vi "Read MotionCorrectionData.vi"(8 "error in (no error)":errorcluster, 10 "ReadSize":u32, 11 "AODAcq in":refnum<class "AODAcq.lvclass">) -> (0 "error out":errorcluster, 2 "MotionCorrectionData":waveform(i32)[](array[waveform]), 3 "AODAcq out":refnum<class "AODAcq.lvclass">)   [LabVIEW 2014, in "AODAcq.lvclass"]
uses:
  AODAcq.lvclass
  AODAcq.lvclass/AODAcq.ctl
  <vilib>/Utility/error.llb/Error Cluster From Error Code.vi
  <vilib>/rvi/errors/niLvFpgaAdjustHostInterfaceError.vi
  HDF5Tools/LabView/Append To Dataset 2D Double.vi
  <vilib>/rvi/interface/nirviMethod/nirviMethod.xnode
  FPGA_Control/AODRef.ctl
  FPGA Bitfiles/AodScanner_FPGATarget_AODControl(FPGA)_TyJc9yYmyGA.lvbitx
  <vilib>/FPGAPlugInAG/PXIe-7965R/niLvFpga_ReadFifo_PXIe-7965R.vi
  <vilib>/rvi/errors/niLvFpgaMergeErrorWithErrorCode.vi
  HDF5Tools/LabView/HDF5Tools.lvlib
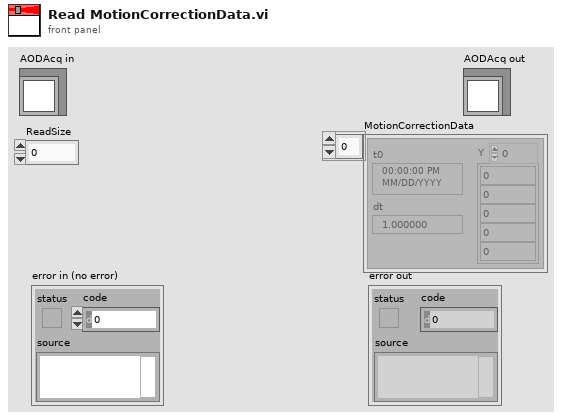
[diagram p1: front panel]
types:
  T1 = typedef "AODRef.ctl" = refnum<k20>
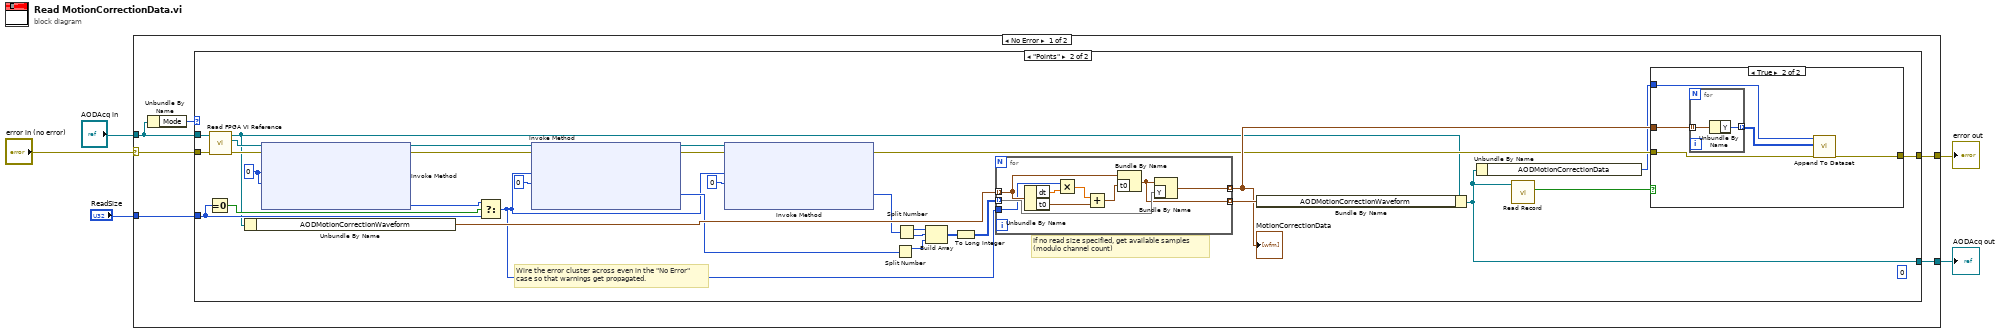
[diagram p0: block diagram]
diagram:
  n1 = case shown="No Error" "error in (no error)" {
    selector: "error in (no error)" -> [w11 w63]
    tunnel: [w8 w63] -> w4
    tunnel: [w9 w62] -> w2
    tunnel: "AODAcq in" -> [w7 w62]
    tunnel: "ReadSize" -> [w10 _]
    frame No Error {
      n2 = Unbundle By Name(w7) -> ("Mode"=w6:enum16{"Idle", "Points", "Volume"})
      n3 = case shown="\"Points\"" w6 {
        tunnel: w7 -> [w13 w44]
        tunnel: w11 -> [w12 w40]
        tunnel: w10 -> [_ w37]
        tunnel: [w13 w32] -> w9
        tunnel: [w12 w31] -> w8
        frame "Idle", Default {
        }
        frame "Points" {
          (unwired) u32 0 ("y")
          w43 = u32 0 ("Number of Elements")
          # "If no read size specified, get available samples \n(modulo channel count)"
          # "Wire the error cluster across even in the \"No Error\"\ncase so that warnings get propagated."
          n4 = Equal To 0?(x=w37) -> (x = 0?=w42:bool)
          n5 = call-dynamic "Read FPGA VI Reference.vi"("error in (no error)"=w40, "AODAcq in"=w44) -> ("error out"=w34:errorcluster, "FPGA VI Reference"=w35:T1, "AODAcq out"=w15:refnum<class "AODAcq.lvclass">)  [unwired: 7 in]
          n6 = Unbundle By Name(w15) -> ("AODMotionCorrectionWaveform"=w39:waveform(i32)[])
          n7 = xnode "Invoke Method"("FPGA VI Reference In"=w35, "error in"=w34, "Number of Elements"=w43, "Timeout (ms)"=w43) -> ("FPGA VI Reference Out"=w27:T1, "error out"=w26:errorcluster, "Elements Remaining"=w36:u32)  [unwired: 1 out]
          n8 = Select(t=w36, s=w42, f=w37) -> (s? t:f=w28:u32)
          n9 = xnode "Invoke Method"("FPGA VI Reference In"=w27, "error in"=w26, "Number of Elements"=w28, "Timeout (ms)"=0) -> ("FPGA VI Reference Out"=w24:T1, "error out"=w25:errorcluster, "Data"=w29:u64[])  [unwired: 1 out]
          n10 = xnode "Invoke Method"("FPGA VI Reference In"=w24, "error in"=w25, "Number of Elements"=w28, "Timeout (ms)"=0) -> ("error out"=w23:errorcluster, "Data"=w21:u64[])  [unwired: 2 out]
          n11 = Split Number(x=w29) -> (hi(x)=w18:u32[])  [unwired: 1 out]
          n12 = Split Number(x=w21) -> (hi(x)=w20:u32[], lo(x)=w19:u32[])
          n13 = Build Array(w20, w19, w18) -> (w17:u32[][])
          n14 = To Long Integer(number=w17) -> (32bit integer=w14:i32[][])
          n15 = for {
            tunnel: w14 -> [w61] mode=indexing
            tunnel: [w60] -> w30 mode=indexing
            tunnel: w39 -> [w56] mode=indexing
            tunnel: w28 -> [w53]
            tunnel: [w54] -> w38 mode=indexing
            n16 = Unbundle By Name(w56) -> ("dt"=w59:dbl, "t0"=w57:timestamp)
            n17 = Multiply(x=w53, y=w59) -> (x*y=w58:dbl)
            n18 = Add(x=w58, y=w57) -> (x+y=w55:timestamp)
            n19 = Bundle By Name(cluster=w56, "t0"=w55) -> (w54:waveform(i32))
            n20 = Bundle By Name(cluster=w54, "Y"=w61) -> (w60:waveform(i32))
          }
          "MotionCorrectionData" <- w30
          n21 = Bundle By Name(cluster=w15, "AODMotionCorrectionWaveform"=w38) -> (w32:refnum<class "AODAcq.lvclass">)
          n22 = Unbundle By Name(w32) -> ("AODMotionCorrectionData"=w16:i32)
          n23 = call-dynamic "Read Record.vi"("AODAcq in"=w32) -> ("Record"=w33:bool)  [unwired: 8 in, 2 out]
          n24 = case shown="True" w33 {
            tunnel: w30 -> [_ w50]
            tunnel: w16 -> [_ w47]
            tunnel: w23 -> [w45 w48]
            tunnel: [w45 w46] -> w31
            frame False {
            }
            frame True {
              n25 = for {
                tunnel: w50 -> [w52] mode=indexing
                tunnel: [w51] -> w49 mode=indexing
                n26 = Unbundle By Name(w52) -> ("Y"=w51:i32[])
              }
              n27 = call-poly "Append To Dataset.vi"("Error in (no error)"=w48, "Data"=w49, "Dataset id in"=w47) -> ("Error out"=w46:errorcluster)  [unwired: 7 in, 1 out]
            }
          }
        }
      }
    }
    frame Error {
    }
  }
  "error out" <- w4
  "AODAcq out" <- w2
